vi "Chronos TDMS Read In Control Values.vi"(7 "Parent":string, 8 "error in (no error)":errorcluster, 9 "Values":variant[](array[variant]), 10 "Properties":string[](array[string]), 11 "Controls":refnum<vi>[](array[refnum])) -> (0 "error out":errorcluster, 1 "All Errors":errorcluster[](array[cluster]))   [LabVIEW 2021]
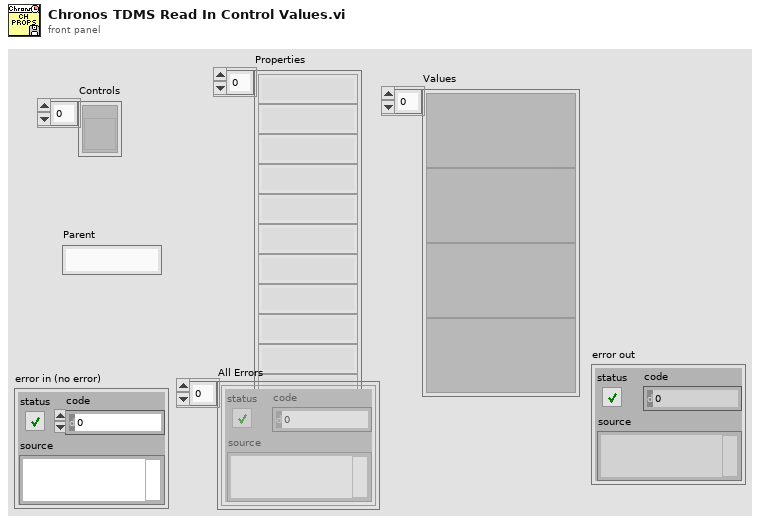
[diagram p1: front panel]
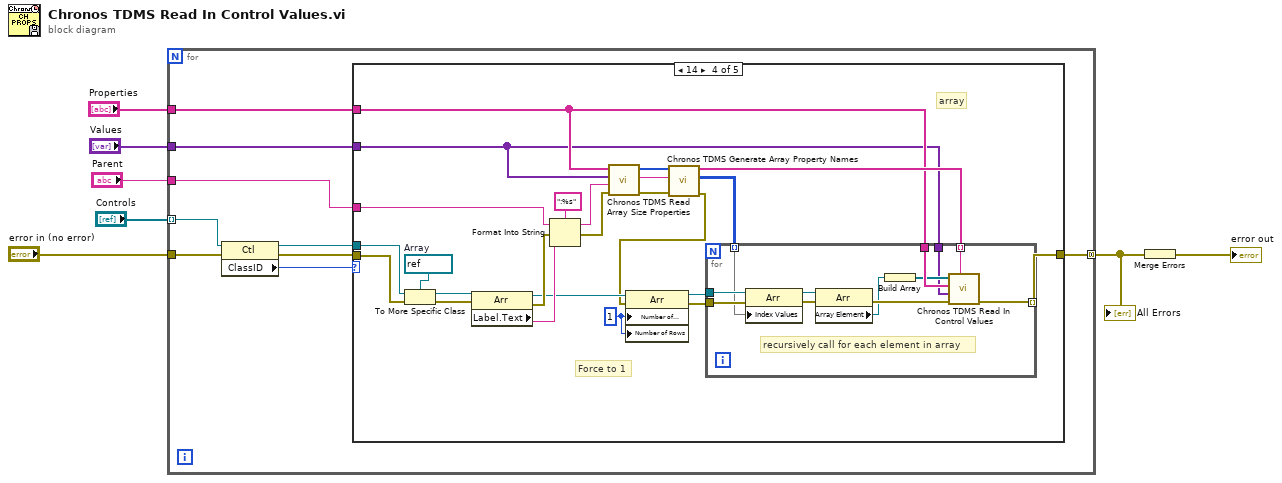
[diagram p0: block diagram]
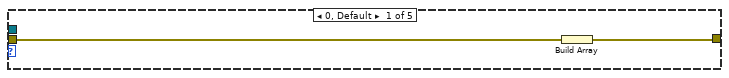
[diagram p2: hidden frame]
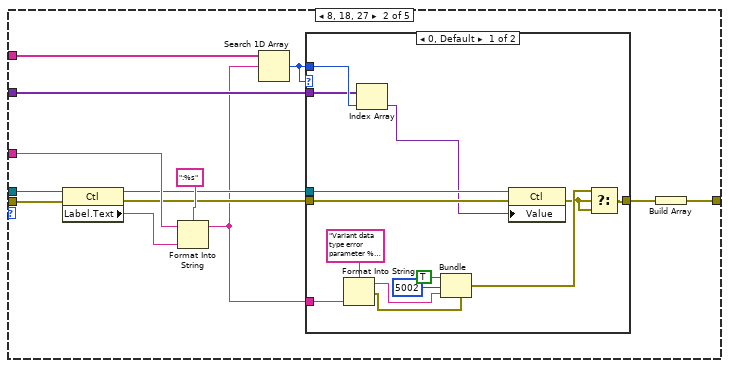
[diagram p3: hidden frame]
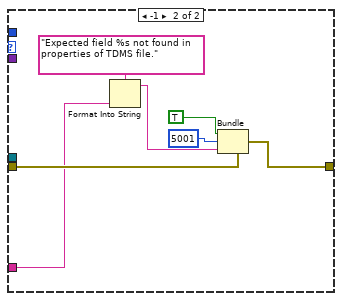
[diagram p4: hidden frame]
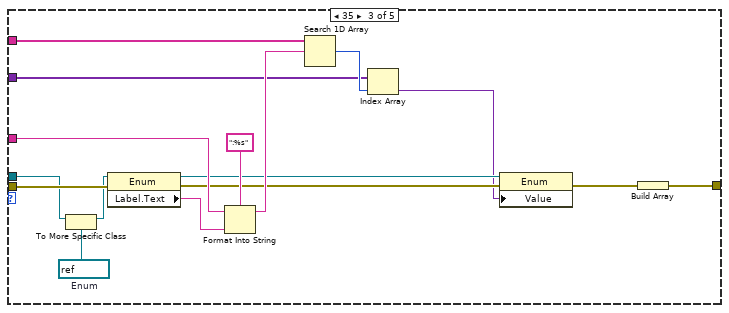
[diagram p5: hidden frame]
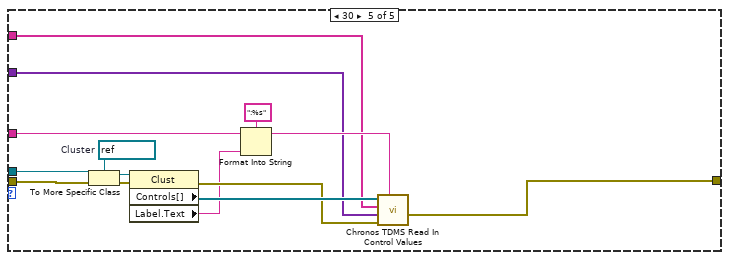
[diagram p6: hidden frame]
diagram:
  n1 = for {
    tunnel: "Controls" -> [w14] mode=indexing
    tunnel: "Parent" -> [w10]
    tunnel: "Properties" -> [w9]
    tunnel: "Values" -> [w8]
    tunnel: "error in (no error)" -> [w16]
    tunnel: [w15] -> w2 mode=concatenating
    n2 = property class="Ctl"(reference=w14, error in=w16) -> (reference out=w12:refnum<vi>, error out=w11:errorcluster, "ClassID"=w13:u32)
    n3 = case shown="14" w13 {
      tunnel: w12 -> [_ w31 w62 w91 w118]
      tunnel: w11 -> [w18 w30 w68 w90 w114]
      tunnel: [w17 w19 w53 w69 w105] -> w15
      tunnel: w10 -> [_ w27 w65 w87 w110]
      tunnel: w9 -> [_ w26 w60 w73 w107]
      tunnel: w8 -> [_ w25 w58 w72 w106]
      frame 0, Default {
        n4 = Build Array(w18) -> (w17:errorcluster[])
      }
      frame 8, 18, 27 {
        n5 = property class="Ctl"(reference=w31, error in=w30) -> (reference out=w24:refnum<vi>, error out=w22:errorcluster, "Label.Text"=w28:string)
        n6 = Format Into String(format string=":%s", initial string=w27, w28) -> (resulting string=w20:string)  [unwired: 1 in, 1 out]
        n7 = Search 1D Array(1D array=w26, element=w20) -> (index of element=w21:i32)  [unwired: 1 in]
        n8 = case shown="0, Default" w21 {
          tunnel: w21 -> [w45 _]
          tunnel: w25 -> [w44 _]
          tunnel: w24 -> [w43 _]
          tunnel: [w34 w51] -> w23
          tunnel: w22 -> [w33 w52]
          tunnel: w20 -> [w41 w49]
          frame 0, Default {
            n9 = Format Into String(format string="Variant data type error parameter %s in TDMS file.", w41) -> (resulting string=w37:string, error out=w40:errorcluster)  [unwired: 2 in]
            n10 = Index Array(array=w44, index=w45) -> (element=w32:variant)
            n11 = Bundle(cluster=w40, "status"=TRUE, "code"=5002, "source"=w37) -> (w36:errorcluster)
            n12 = property class="Ctl"(reference=w43, error in=w33, "Value"=w32) -> (error out=w35:errorcluster)  [unwired: 1 out]
            n13 = Select(t=w36, s=w35, f=w35) -> (s? t:f=w34:errorcluster)
          }
          frame -1 {
            n14 = Format Into String(format string="Expected field %s not found in properties of TDMS file.", w49) -> (resulting string=w48:string)  [unwired: 2 in, 1 out]
            n15 = Bundle(cluster=w52, "status"=TRUE, "code"=5001, "source"=w48) -> (w51:errorcluster)
          }
        }
        n16 = Build Array(w23) -> (w19:errorcluster[])
      }
      frame 35 {
        w64 = refnum<vi> refnum  # Enum
        n17 = To More Specific Class(target class=w64, reference=w62) -> (specific class reference=w63:refnum<vi>)  [unwired: 1 in, 1 out]
        n18 = property class="Enum"(reference=w63, error in=w68) -> (reference out=w56:refnum<vi>, error out=w55:errorcluster, "Label.Text"=w66:string)
        n19 = Format Into String(format string=":%s", initial string=w65, w66) -> (resulting string=w59:string)  [unwired: 1 in, 1 out]
        n20 = Search 1D Array(1D array=w60, element=w59) -> (index of element=w61:i32)  [unwired: 1 in]
        n21 = Index Array(array=w58, index=w61) -> (element=w54:variant)
        n22 = property class="Enum"(reference=w56, error in=w55, "Value"=w54) -> (error out=w57:errorcluster)  [unwired: 1 out]
        n23 = Build Array(w57) -> (w53:errorcluster[])
      }
      frame 14 {
        w78 = u32 1 ("Number of Columns")
        w92 = refnum<vi> refnum  # Array
        # "Force to 1"
        # "array"
        n24 = To More Specific Class(target class=w92, reference=w91, error in=w90) -> (specific class reference=w89:refnum<vi>, error out=w86:errorcluster)
        n25 = property class="Arr"(reference=w89, error in=w86) -> (reference out=w77:refnum<vi>, error out=w85:errorcluster, "Label.Text"=w81:string)
        n26 = Format Into String(format string=":%s", initial string=w87, error in=w85, w81) -> (resulting string=w79:string, error out=w84:errorcluster)
        n27 = call "Chronos TDMS Read Array Size Properties.vi"("error in (no error)"=w84, "Label"=w79, "Values"=w72, "Properties"=w73) -> ("error out"=w80:errorcluster, "Label dup"=w82:string, "Array Dimensions"=w83:i32[])  [unwired: 5 in]
        n28 = call "Chronos TDMS Generate Array Property Names.vi"("error in (no error)"=w80, "Label"=w82, "Array Dimensions"=w83) -> ("error out"=w71:errorcluster, "Indecies"=w70:i32[][], "Array Property Names"=w74:string[])  [unwired: 6 in]
        n29 = property class="Arr"(reference=w77, error in=w71, "Number of Columns"=w78, "Number of Rows"=w78) -> (reference out=w75:refnum<vi>, error out=w76:errorcluster)
        n30 = for {
          tunnel: w75 -> [w103]
          tunnel: w73 -> [w99]
          tunnel: w74 -> [w97] mode=indexing
          tunnel: w76 -> [w102]
          tunnel: [w96] -> w69 mode=indexing
          tunnel: w72 -> [w94]
          tunnel: w70 -> [w93] mode=indexing
          # "recursively call for each element in array"
          n31 = property class="Arr"(reference=w103, error in=w102, "Index Values"=w93) -> (reference out=w104:refnum<vi>, error out=w101:errorcluster)
          n32 = property class="Arr"(reference=w104, error in=w101) -> (error out=w100:errorcluster, "Array Element"=w95:refnum<vi>)  [unwired: 1 out]
          n33 = Build Array(w95) -> (w98:refnum<vi>[])
          n34 = call "Chronos TDMS Read In Control Values.vi"("Parent"=w97, "error in (no error)"=w100, "Values"=w94, "Properties"=w99, "Controls"=w98) -> ("error out"=w96:errorcluster)  [unwired: 5 in, 1 out]
        }
      }
      frame 30 {
        w117 = refnum<vi> refnum  # Cluster
        n35 = To More Specific Class(target class=w117, reference=w118, error in=w114) -> (specific class reference=w116:refnum<vi>, error out=w115:errorcluster)
        n36 = property class="Clust"(reference=w116, error in=w115) -> (error out=w112:errorcluster, "Controls[]"=w113:refnum<vi>[], "Label.Text"=w109:string)  [unwired: 1 out]
        n37 = Format Into String(format string=":%s", initial string=w110, w109) -> (resulting string=w108:string)  [unwired: 1 in, 1 out]
        n38 = call "Chronos TDMS Read In Control Values.vi"("Parent"=w108, "error in (no error)"=w112, "Values"=w106, "Properties"=w107, "Controls"=w113) -> ("All Errors"=w105:errorcluster[])  [unwired: 5 in, 1 out]
      }
    }
  }
  "All Errors" <- w2
  n39 = Merge Errors(w2) -> (→"error out":errorcluster)
